vi "战舰+敌机玉石俱焚.vi"() -> ()   [LabVIEW 2018]
panel:
  out "战舰爆炸":picture
  out "血量":dbl
  out "战舰血量":T1 scale=0.0..100.0
  out "敌机爆炸":picture
  in  "敌机数量":dbl
  in  "敌机速度":dbl
  out "敌机":picture
  out "按键":dbl
  out "战舰":T2
  out "激光武器1":T3
  out "激光武器 2":T3
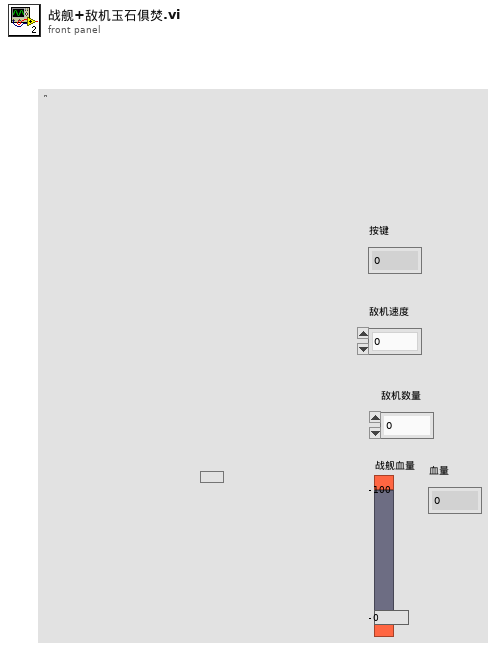
[diagram p1: front panel]
types:
  T1 = typedef "战列巡洋舰_血条.ctl" = dbl
  T2 = typedef "战列巡洋舰.ctl" = picture
  T3 = typedef "战列巡洋舰_激光武器.ctl" = picture
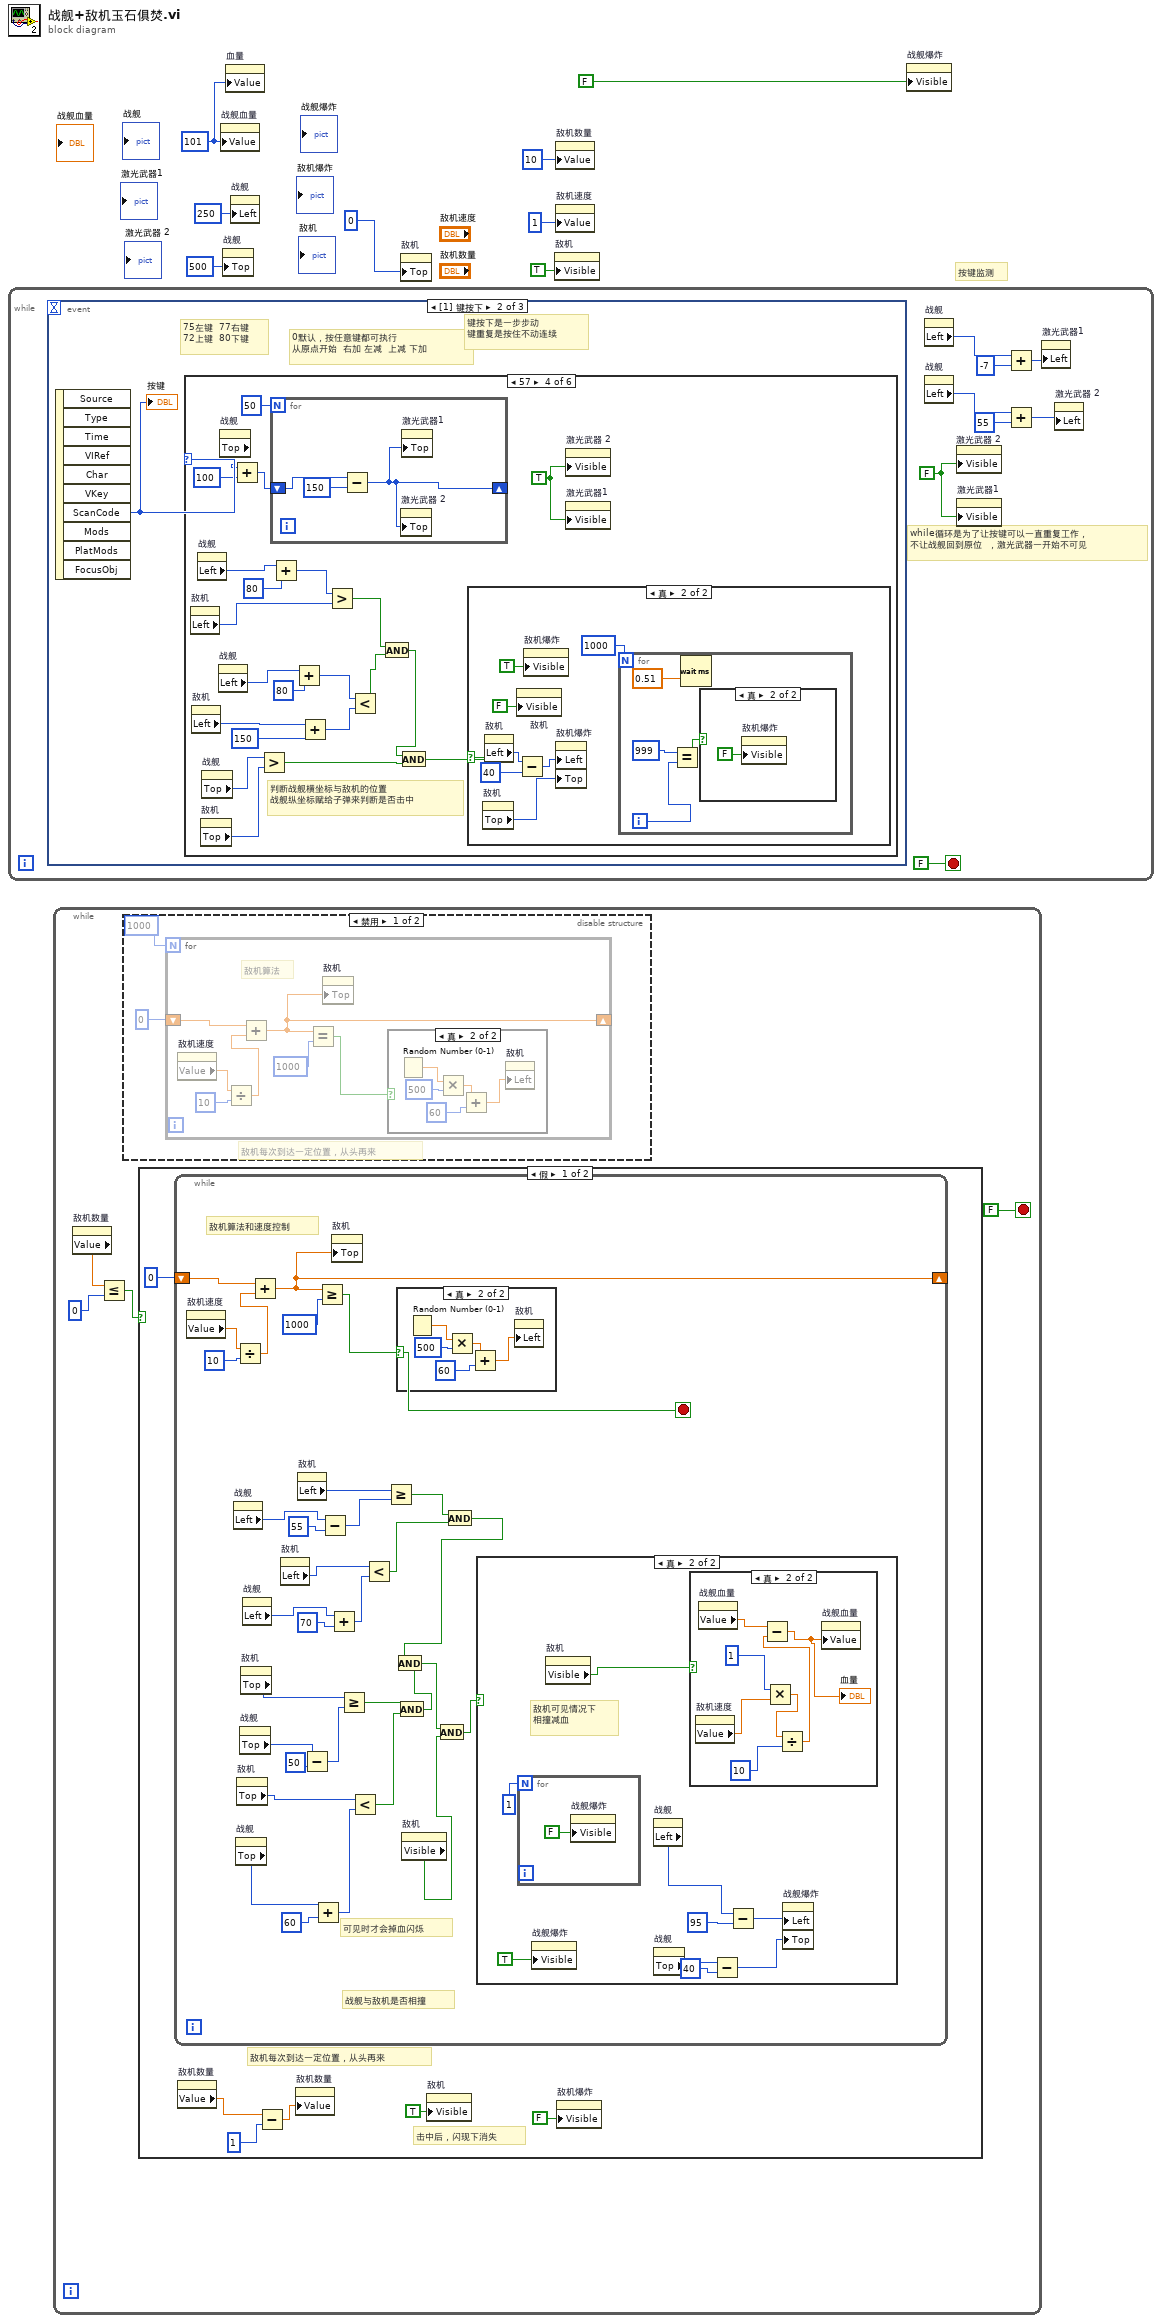
[diagram p0: block diagram]
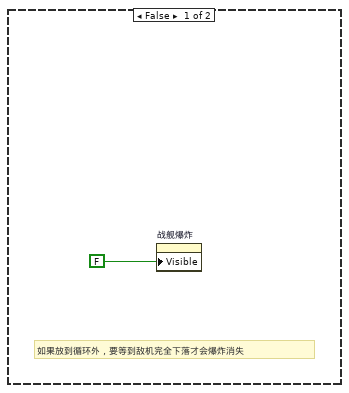
[diagram p2: hidden frame]
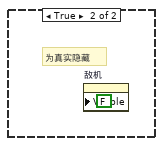
[diagram p5: hidden frame]
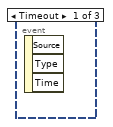
[diagram p8: hidden frame]
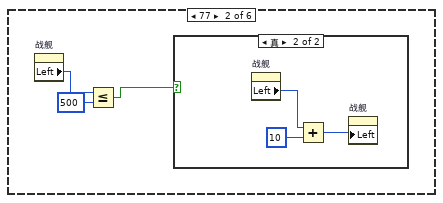
[diagram p10: hidden frame]
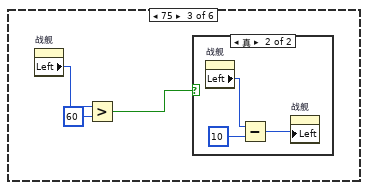
[diagram p12: hidden frame]
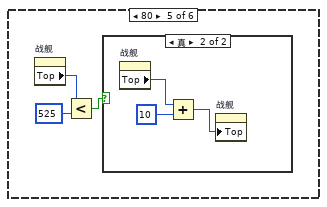
[diagram p16: hidden frame]
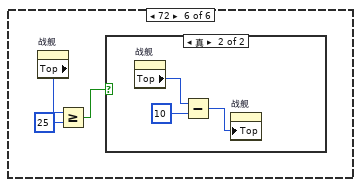
[diagram p18: hidden frame]
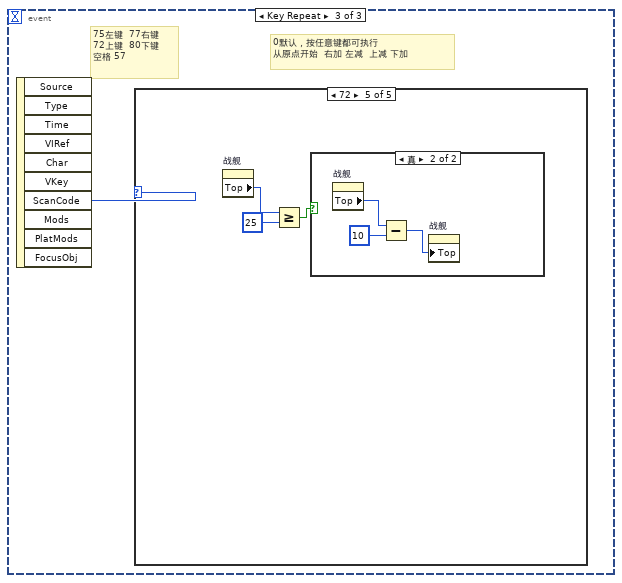
[diagram p20: hidden frame]
diagram:
  w2 = 101
  # "按键监测"
  n1 = while {
    stop <- FALSE stop-if-true
    w9 = FALSE
    # "while循环是为了让按键可以一直重复工作，\n不让战舰回到原位  ，激光武器一开始不可见"
    n2 = event shown="[1] 键按下" {
      selector: _ -> [_ _ _]
      dyn-events: _ -> [_ _ _]
      timeout: _ -> [_ _ _]
      event Timeout {
        n3 = event-data() -> ()  [unwired: 1 in, 3 out]
      }
      event Key Down {
        # "键按下是一步步动\n键重复是按住不动连续"
        # "75左键  77右键\n72上键  80下键"
        # "0默认，按任意键都可执行\n从原点开始  右加 左减  上减 下加"
        n4 = event-data() -> ("ScanCode"=w17:i16)  [unwired: 1 in, 9 out]
        "按键" <- w17
        n5 = case shown="57" w17 {
          frame 0, Default {
          }
          frame 77 {
            n6 = property on="战舰" class="Pict (严格)"() -> ("Left"=w20:i32)  [unwired: 2 in, 2 out]
            n7 = Less Or Equal?(x=w20, y=500) -> (x <= y?=w18:bool)
            n8 = case shown="真" w18 {
              frame False {
              }
              frame True {
                n9 = property on="战舰" class="Pict (严格)"() -> ("Left"=w22:i32)  [unwired: 2 in, 2 out]
                n10 = Add(x=w22, y=10) -> (x+y=w23:i32)
                n11 = property on="战舰" class="Pict (严格)"("Left"=w23) -> ()  [unwired: 2 in, 2 out]
              }
            }
          }
          frame 75 {
            n12 = property on="战舰" class="Pict (严格)"() -> ("Left"=w26:i32)  [unwired: 2 in, 2 out]
            n13 = Greater?(x=w26, y=60) -> (0:w24:bool)
            n14 = case shown="真" w24 {
              frame False {
              }
              frame True {
                n15 = property on="战舰" class="Pict (严格)"() -> ("Left"=w28:i32)  [unwired: 2 in, 2 out]
                n16 = Subtract(x=w28, y=10) -> (x-y=w29:i32)
                n17 = property on="战舰" class="Pict (严格)"("Left"=w29) -> ()  [unwired: 2 in, 2 out]
              }
            }
          }
          frame 57 {
            w47 = TRUE
            # "判断战舰横坐标与敌机的位置\n战舰纵坐标赋给子弹来判断是否击中"
            n18 = property on="敌机" class="Pict"() -> ("Left"=w44:i32)  [unwired: 2 in, 2 out]
            n19 = property on="敌机" class="Pict"() -> ("Left"=w37:i32)  [unwired: 2 in, 2 out]
            n20 = property on="战舰" class="Pict (严格)"() -> ("Left"=w46:i32)  [unwired: 2 in, 2 out]
            n21 = property on="敌机" class="Pict"() -> ("Top"=w30:i32)  [unwired: 2 in, 2 out]
            n22 = property on="战舰" class="Pict (严格)"() -> ("Top"=w31:i32)  [unwired: 2 in, 2 out]
            n23 = property on="战舰" class="Pict (严格)"() -> ("Left"=w39:i32)  [unwired: 2 in, 2 out]
            n24 = property on="战舰" class="Pict (严格)"() -> ("Top"=w50:i32)  [unwired: 2 in, 2 out]
            n25 = Add(x=w50, y=100) -> (x+y=w48:i32)
            n26 = Greater?(x=w31, y=w30) -> (0:w33:bool)
            n27 = for {
              N: 50 -> [_]
              shift-right: [w64] -> _
              shift-left: w48 -> [w66]
              n28 = Subtract(x=w66, y=150) -> (x-y=w64:i32)
              n29 = property on="激光武器 2" class="Pict (严格)"("Top"=w64) -> ()  [unwired: 2 in, 2 out]
              n30 = property on="激光武器1" class="Pict (严格)"("Top"=w64) -> ()  [unwired: 2 in, 2 out]
            }
            n31 = Add(x=w46, y=80) -> (x+y=w43:i32)
            n32 = Add(x=w39, y=80) -> (x+y=w41:i32)
            n33 = Add(x=w37, y=150) -> (x+y=w36:i32)
            n34 = Greater?(x=w43, y=w44) -> (0:w42:bool)
            n35 = Less?(x=w41, y=w36) -> (x < y?=w38:bool)
            n36 = And(x=w42, y=w38) -> (x .and. y?=w34:bool)
            n37 = And(x=w34, y=w33) -> (x .and. y?=w32:bool)
            n38 = case shown="真" w32 {
              frame False {
              }
              frame True {
                n39 = property on="敌机" class="Pict"() -> ("Top"=w56:i32)  [unwired: 2 in, 2 out]
                n40 = property on="敌机" class="Pict"() -> ("Left"=w54:i32)  [unwired: 2 in, 2 out]
                n41 = property on="敌机" class="Pict"("Visible"=FALSE ("可见")) -> ()  [unwired: 2 in, 2 out]
                n42 = Subtract(x=w54, y=40) -> (x-y=w53:i32)
                n43 = property on="敌机爆炸" class="Pict"("Visible"=TRUE ("可见")) -> ()  [unwired: 2 in, 2 out]
                n44 = property on="敌机爆炸" class="Pict"("Left"=w53, "Top"=w56) -> ()  [unwired: 2 in, 2 out]
                n45 = for {
                  N: 1000 -> [_]
                  i -> [w61]
                  n46 = Equal?(x=999, y=w61) -> (x = y?=w62:bool)
                  n47 = Wait (ms)(milliseconds to wait=0.51) -> ()  [unwired: 1 out]
                  n48 = case shown="真" w62 {
                    frame False {
                    }
                    frame True {
                      n49 = property on="敌机爆炸" class="Pict"("Visible"=FALSE ("可见")) -> ()  [unwired: 2 in, 2 out]
                    }
                  }
                }
              }
            }
            n50 = property on="激光武器 2" class="Pict (严格)"("Visible"=w47) -> ()  [unwired: 2 in, 2 out]
            n51 = property on="激光武器1" class="Pict (严格)"("Visible"=w47) -> ()  [unwired: 2 in, 2 out]
          }
          frame 80 {
            n52 = property on="战舰" class="Pict (严格)"() -> ("Top"=w69:i32)  [unwired: 2 in, 2 out]
            n53 = Less?(x=w69, y=525) -> (x < y?=w67:bool)
            n54 = case shown="真" w67 {
              frame False {
              }
              frame True {
                n55 = property on="战舰" class="Pict (严格)"() -> ("Top"=w71:i32)  [unwired: 2 in, 2 out]
                n56 = Add(x=w71, y=10) -> (x+y=w70:i32)
                n57 = property on="战舰" class="Pict (严格)"("Top"=w70) -> ()  [unwired: 2 in, 2 out]
              }
            }
          }
          frame 72 {
            n58 = property on="战舰" class="Pict (严格)"() -> ("Top"=w75:i32)  [unwired: 2 in, 2 out]
            n59 = Greater Or Equal?(x=w75, y=25) -> (x >= y?=w74:bool)
            n60 = case shown="真" w74 {
              frame False {
              }
              frame True {
                n61 = property on="战舰" class="Pict (严格)"() -> ("Top"=w78:i32)  [unwired: 2 in, 2 out]
                n62 = Subtract(x=w78, y=10) -> (x-y=w77:i32)
                n63 = property on="战舰" class="Pict (严格)"("Top"=w77) -> ()  [unwired: 2 in, 2 out]
              }
            }
          }
        }
      }
      event Key Repeat {
        # "75左键  77右键\n72上键  80下键\n空格 57"
        # "0默认，按任意键都可执行\n从原点开始  右加 左减  上减 下加"
        n64 = event-data() -> ("ScanCode"=w79:i16)  [unwired: 1 in, 9 out]
        n65 = case shown="72" w79 {
          frame 0, Default {
          }
          frame 77 {
            n66 = property on="战舰" class="Pict (严格)"() -> ("Left"=w82:i32)  [unwired: 2 in, 2 out]
            n67 = Less Or Equal?(x=w82, y=500) -> (x <= y?=w81:bool)
            n68 = case shown="真" w81 {
              frame False {
              }
              frame True {
                n69 = property on="战舰" class="Pict (严格)"() -> ("Left"=w84:i32)  [unwired: 2 in, 2 out]
                n70 = Add(x=w84, y=10) -> (x+y=w85:i32)
                n71 = property on="战舰" class="Pict (严格)"("Left"=w85) -> ()  [unwired: 2 in, 2 out]
              }
            }
          }
          frame 75 {
            n72 = property on="战舰" class="Pict (严格)"() -> ("Left"=w88:i32)  [unwired: 2 in, 2 out]
            n73 = Greater Or Equal?(x=w88, y=25) -> (x >= y?=w87:bool)
            n74 = case shown="真" w87 {
              frame False {
              }
              frame True {
                n75 = property on="战舰" class="Pict (严格)"() -> ("Left"=w91:i32)  [unwired: 2 in, 2 out]
                n76 = Subtract(x=w91, y=10) -> (x-y=w90:i32)
                n77 = property on="战舰" class="Pict (严格)"("Left"=w90) -> ()  [unwired: 2 in, 2 out]
              }
            }
          }
          frame 80 {
            n78 = property on="战舰" class="Pict (严格)"() -> ("Top"=w94:i32)  [unwired: 2 in, 2 out]
            n79 = Less Or Equal?(x=w94, y=525) -> (x <= y?=w93:bool)
            n80 = case shown="真" w93 {
              frame False {
              }
              frame True {
                n81 = property on="战舰" class="Pict (严格)"() -> ("Top"=w96:i32)  [unwired: 2 in, 2 out]
                n82 = Add(x=w96, y=10) -> (x+y=w95:i32)
                n83 = property on="战舰" class="Pict (严格)"("Top"=w95) -> ()  [unwired: 2 in, 2 out]
              }
            }
          }
          frame 72 {
            n84 = property on="战舰" class="Pict (严格)"() -> ("Top"=w100:i32)  [unwired: 2 in, 2 out]
            n85 = Greater Or Equal?(x=w100, y=25) -> (x >= y?=w99:bool)
            n86 = case shown="真" w99 {
              frame False {
              }
              frame True {
                n87 = property on="战舰" class="Pict (严格)"() -> ("Top"=w103:i32)  [unwired: 2 in, 2 out]
                n88 = Subtract(x=w103, y=10) -> (x-y=w102:i32)
                n89 = property on="战舰" class="Pict (严格)"("Top"=w102) -> ()  [unwired: 2 in, 2 out]
              }
            }
          }
        }
      }
    }
    n90 = property on="战舰" class="Pict (严格)"() -> ("Left"=w15:i32)  [unwired: 2 in, 2 out]
    n91 = property on="战舰" class="Pict (严格)"() -> ("Left"=w11:i32)  [unwired: 2 in, 2 out]
    n92 = property on="激光武器 2" class="Pict (严格)"("Visible"=w9) -> ()  [unwired: 2 in, 2 out]
    n93 = property on="激光武器1" class="Pict (严格)"("Visible"=w9) -> ()  [unwired: 2 in, 2 out]
    n94 = Add(x=w15, y=-7) -> (x+y=w14:i32)
    n95 = Add(x=w11, y=55) -> (x+y=w10:i32)
    n96 = property on="激光武器1" class="Pict (严格)"("Left"=w14) -> ()  [unwired: 2 in, 2 out]
    n97 = property on="激光武器 2" class="Pict (严格)"("Left"=w10) -> ()  [unwired: 2 in, 2 out]
  }
  n98 = while {
    stop <- FALSE stop-if-true
    n99 = property on="敌机数量" class="DigNum (严格)"() -> ("Value"=w106:dbl)  [unwired: 2 in, 2 out]
    n100 = Less Or Equal?(x=w106, y=0) -> (x <= y?=w105:bool)
    n101 = disable-structure shown="禁用" {
      frame Disabled {
        # "敌机每次到达一定位置，从头再来"
        n102 = for {
          N: 1000 -> [_]
          shift-right: [w175] -> _
          shift-left: 0 -> [w178]
          # "敌机算法"
          n103 = property on="敌机速度" class="DigNum (严格)"() -> ("Value"=w174:dbl)  [unwired: 2 in, 2 out]
          n104 = Divide(x=w174, y=10) -> (x/y=w173:dbl)
          n105 = Add(x=w178, y=w173) -> (x+y=w175:dbl)
          n106 = Equal?(x=w175, y=1000) -> (x = y?=w176:bool)
          n107 = property on="敌机" class="Pict"("Top"=w175) -> ()  [unwired: 2 in, 2 out]
          n108 = case shown="真" w176 {
            frame False {
            }
            frame True {
              n109 = Random Number (0-1)() -> (number: 0 to 1=w183:dbl)
              n110 = Multiply(x=w183, y=500) -> (x*y=w181:dbl)
              n111 = Add(x=w181, y=60) -> (x+y=w180:dbl)
              n112 = property on="敌机" class="Pict"("Left"=w180) -> ()  [unwired: 2 in, 2 out]
            }
          }
        }
      }
      frame Enabled {
      }
    }
    n113 = case shown="假" w105 {
      frame False {
        # "击中后，闪现下消失"
        # "敌机每次到达一定位置，从头再来"
        n114 = while {
          shift-right: [w143] -> _
          shift-left: 0 -> [w145]
          stop <- w139 stop-if-true
          # "可见时才会掉血闪烁"
          # "战舰与敌机是否相撞"
          # "敌机算法和速度控制"
          n115 = property on="敌机速度" class="DigNum (严格)"() -> ("Value"=w142:dbl)  [unwired: 2 in, 2 out]
          n116 = property on="战舰" class="Pict (严格)"() -> ("Left"=w137:i32)  [unwired: 2 in, 2 out]
          n117 = Divide(x=w142, y=10) -> (x/y=w141:dbl)
          n118 = property on="战舰" class="Pict (严格)"() -> ("Top"=w121:i32)  [unwired: 2 in, 2 out]
          n119 = property on="敌机" class="Pict"() -> ("Top"=w120:i32)  [unwired: 2 in, 2 out]
          n120 = property on="战舰" class="Pict (严格)"() -> ("Top"=w127:i32)  [unwired: 2 in, 2 out]
          n121 = property on="敌机" class="Pict"() -> ("Top"=w128:i32)  [unwired: 2 in, 2 out]
          n122 = property on="战舰" class="Pict (严格)"() -> ("Left"=w131:i32)  [unwired: 2 in, 2 out]
          n123 = Add(x=w145, y=w141) -> (x+y=w143:dbl)
          n124 = property on="敌机" class="Pict"() -> ("Left"=w133:i32)  [unwired: 2 in, 2 out]
          n125 = property on="敌机" class="Pict"() -> ("Left"=w138:i32)  [unwired: 2 in, 2 out]
          n126 = Subtract(x=w127, y=50) -> (x-y=w125:i32)
          n127 = Add(x=w121, y=60) -> (x+y=w123:i32)
          n128 = Greater Or Equal?(x=w143, y=1000) -> (x >= y?=w139:bool)
          n129 = Subtract(x=w137, y=55) -> (x-y=w136:i32)
          n130 = Add(x=w131, y=70) -> (x+y=w130:i32)
          n131 = property on="敌机" class="Pict"("Top"=w143) -> ()  [unwired: 2 in, 2 out]
          n132 = Greater Or Equal?(x=w128, y=w125) -> (x >= y?=w119:bool)
          n133 = Less?(x=w120, y=w123) -> (x < y?=w118:bool)
          n134 = Less?(x=w133, y=w130) -> (x < y?=w129:bool)
          n135 = Greater Or Equal?(x=w138, y=w136) -> (x >= y?=w134:bool)
          n136 = case shown="真" w139 {
            frame False {
            }
            frame True {
              n137 = Random Number (0-1)() -> (number: 0 to 1=w168:dbl)
              n138 = Multiply(x=w168, y=500) -> (x*y=w166:dbl)
              n139 = Add(x=w166, y=60) -> (x+y=w165:dbl)
              n140 = property on="敌机" class="Pict"("Left"=w165) -> ()  [unwired: 2 in, 2 out]
            }
          }
          n141 = And(x=w119, y=w118) -> (x .and. y?=w117:bool)
          n142 = property on="敌机" class="Pict"() -> ("Visible"=w115:bool)  [unwired: 2 in, 2 out]
          n143 = And(x=w134, y=w129) -> (x .and. y?=w124:bool)
          n144 = And(x=w124, y=w117) -> (x .and. y?=w116:bool)
          n145 = And(x=w116, y=w115) -> (x .and. y?=w114:bool)
          n146 = case shown="真" w114 {
            frame False {
              # "如果放到循环外，要等到敌机完全下落才会爆炸消失"
              n147 = property on="战舰爆炸" class="Pict"("Visible"=FALSE ("可见")) -> ()  [unwired: 2 in, 2 out]
            }
            frame True {
              # "敌机可见情况下\n相撞减血"
              n148 = for {
                N: 1 -> [_]
                n149 = property on="战舰爆炸" class="Pict"("Visible"=FALSE ("可见")) -> ()  [unwired: 2 in, 2 out]
              }
              n150 = property on="战舰爆炸" class="Pict"("Visible"=TRUE ("可见")) -> ()  [unwired: 2 in, 2 out]
              n151 = property on="敌机" class="Pict"() -> ("Visible"=w155:bool)  [unwired: 2 in, 2 out]
              n152 = property on="战舰" class="Pict (严格)"() -> ("Left"=w153:i32)  [unwired: 2 in, 2 out]
              n153 = property on="战舰" class="Pict (严格)"() -> ("Top"=w150:i32)  [unwired: 2 in, 2 out]
              n154 = case shown="真" w155 {
                frame False {
                }
                frame True {
                  n155 = property on="敌机速度" class="DigNum (严格)"() -> ("Value"=w162:dbl)  [unwired: 2 in, 2 out]
                  n156 = property on="战舰血量" class="Slide (严格)"() -> ("Value"=w163:T1)  [unwired: 2 in, 2 out]
                  n157 = Multiply(x=1, y=w162) -> (x*y=w161:dbl)
                  n158 = Divide(x=w161, y=10) -> (x/y=w158:dbl)
                  n159 = Subtract(x=w163, y=w158) -> (x-y=w157:T1)
                  "血量" <- w157
                  n160 = property on="战舰血量" class="Slide (严格)"("Value"=w157) -> ()  [unwired: 2 in, 2 out]
                }
              }
              n161 = Subtract(x=w150, y=40) -> (x-y=w148:i32)
              n162 = Subtract(x=w153, y=95) -> (x-y=w151:i32)
              n163 = property on="战舰爆炸" class="Pict"("Left"=w151, "Top"=w148) -> ()  [unwired: 2 in, 2 out]
            }
          }
        }
        n164 = property on="敌机数量" class="DigNum (严格)"() -> ("Value"=w111:dbl)  [unwired: 2 in, 2 out]
        n165 = Subtract(x=w111, y=1) -> (x-y=w112:dbl)
        n166 = property on="敌机数量" class="DigNum (严格)"("Value"=w112) -> ()  [unwired: 2 in, 2 out]
        n167 = property on="敌机" class="Pict"("Visible"=TRUE ("可见")) -> ()  [unwired: 2 in, 2 out]
        n168 = property on="敌机爆炸" class="Pict"("Visible"=FALSE ("可见")) -> ()  [unwired: 2 in, 2 out]
      }
      frame True {
        # "为真实隐藏"
        n169 = property on="敌机" class="Pict"("Visible"=FALSE ("可见")) -> ()  [unwired: 2 in, 2 out]
      }
    }
  }
  n170 = property on="战舰血量" class="Slide (严格)"("Value"=w2) -> ()  [unwired: 2 in, 2 out]
  n171 = property on="战舰" class="Pict (严格)"("Top"=500 ("位置:置顶")) -> ()  [unwired: 2 in, 2 out]
  n172 = property on="血量" class="DigNum (严格)"("Value"=w2) -> ()  [unwired: 2 in, 2 out]
  n173 = property on="战舰" class="Pict (严格)"("Left"=250 ("位置:居左")) -> ()  [unwired: 2 in, 2 out]
  n174 = property on="敌机" class="Pict"("Top"=0) -> ()  [unwired: 2 in, 2 out]
  n175 = property on="敌机" class="Pict"("Visible"=TRUE ("可见")) -> ()  [unwired: 2 in, 2 out]
  n176 = property on="敌机数量" class="DigNum (严格)"("Value"=10) -> ()  [unwired: 2 in, 2 out]
  n177 = property on="敌机速度" class="DigNum (严格)"("Value"=1) -> ()  [unwired: 2 in, 2 out]
  n178 = property on="战舰爆炸" class="Pict"("Visible"=FALSE ("可见")) -> ()  [unwired: 2 in, 2 out]
